vi "Delete temp folders.vi"(8 "error in (no error)":errorcluster, 11 "a3Di Stations":enum16{"APG", "Inspection", "Diagnostic"}[](array[ring])) -> (0 "error out":errorcluster)   [LabVIEW 2013, in "Manipulate IPF.lvlib"]
uses:
  <vilib>/Utility/sysdir.llb/System Directory Type.ctl
  Manipulate IPF.lvlib
panel:
  out "Temp folders deleted":path[](array[path])
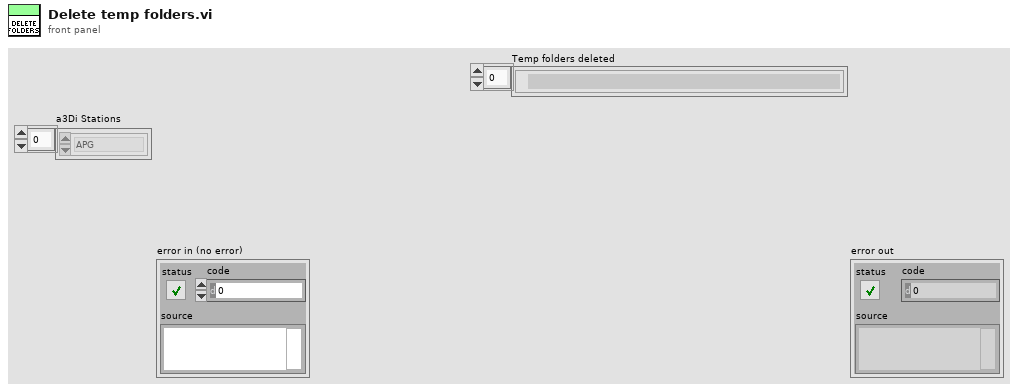
[diagram p1: front panel]
types:
  T1 = typedef "System Directory Type.ctl" = i32
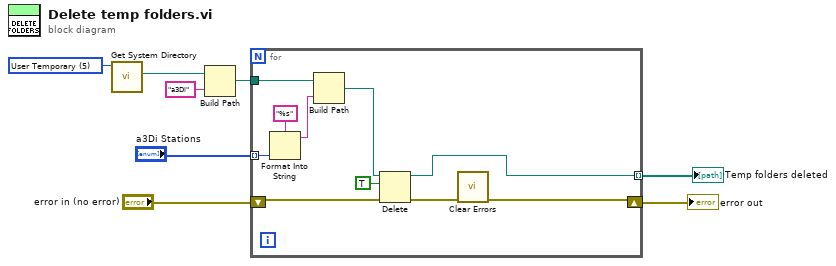
[diagram p0: block diagram]
diagram:
  w8 = T1 5 items=["User Home"=0, "User Desktop"=1, "User Documents"=2, "User Application Data"=3, "User Preferences"=4, "User Temporary"=5, "Public Documents"=6, "Public Application Data"=7, "Public Preferences"=8, "Public Cache"=13, "System Core Libraries"=9, "System Installed Libraries"=10, "Application Files"=11, "Boot Volume Root"=12] ("system directory type")
  n1 = call <vilib>:"Get System Directory.vi"("system directory type"=w8) -> ("system directory"=w5:path)  [unwired: 10 in]
  n2 = Build Path(base path=w5, name or relative path="a3Di") -> (appended path=w4:path)
  n3 = for {
    shift-right: [w10] -> w7
    shift-left: "error in (no error)" -> [w12]
    tunnel: "a3Di Stations" -> [w17] mode=indexing
    tunnel: w4 -> [w18]
    tunnel: [w9] -> w2 mode=indexing
    n4 = Format Into String(format string="%s", w17) -> (resulting string=w16:string)  [unwired: 2 in, 1 out]
    n5 = Build Path(base path=w18, name or relative path=w16) -> (appended path=w13:path)
    n6 = Delete(path (use dialog)=w13, entire hierarchy (F)=TRUE, error in=w12) -> (deleted path=w9:path, error out=w11:errorcluster)  [unwired: 2 in, 1 out]
    n7 = call <vilib>:"Clear Errors.vi"("error in (no error)"=w11) -> ("error out"=w10:errorcluster)  [unwired: 6 in]
  }
  "error out" <- w7
  "Temp folders deleted" <- w2
